vi "Set Calibration (SubVI).vi"(11 "Calibration in":T1 {"Max Current A" format="%#_g mA"; "Max Current B" format="%#_g mA"; "UCL A" format="%#_g mA"; "LCL A" format="%#_g mA"; "UCL B" format="%#_g mA"; "LCL B" format="%#_g mA"}) -> (1 "Array":string[](array[string]))   [LabVIEW 2015]
uses:
  03 Type Def & Global/Calibration.ctl
  <vilib>/Utility/miscctls.llb/LVPointTypeDef.ctl
panel:
  in  "Cancel Button":bool
  in  "OK Button":bool
  in  "Calibration":T1={"Max Current A"=290.0, "Max Current B"=290.0, "UCL A"=290.0, "UCL B"=290.0, "LCL A"=0.0, "LCL B"=0.0} {"Max Current A" format="%#_g mA"; "Max Current B" format="%#_g mA"; "UCL A" format="%#_g mA"; "LCL A" format="%#_g mA"; "UCL B" format="%#_g mA"; "LCL B" format="%#_g mA"}
  # "Please change the calbration values as needed"
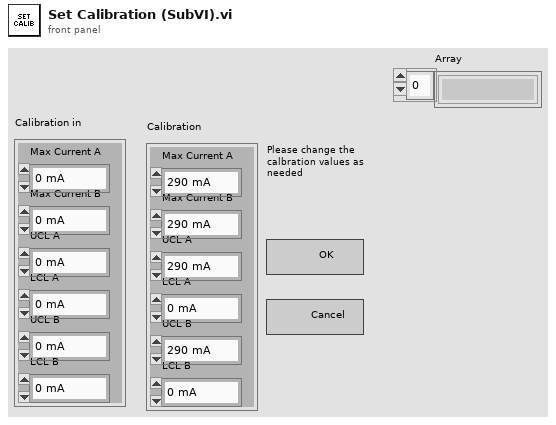
[diagram p1: front panel]
types:
  T1 = typedef "Calibration.ctl" = cluster{"Max Current A":dbl, "Max Current B":dbl, "UCL A":dbl, "UCL B":dbl, "LCL A":dbl, "LCL B":dbl}
  T2 = typedef "LVPointTypeDef.ctl" = cluster{"Horizontal":i16, "Vertical":i16}
  T3 = cluster{"Max Current A":bool, "Max Current B":bool, "UCL A":bool, "UCL B":bool, "LCL A":bool, "LCL B":bool}
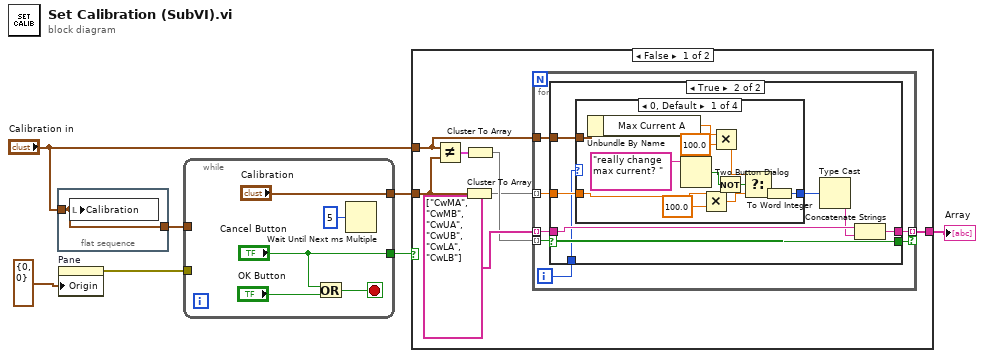
[diagram p0: block diagram]
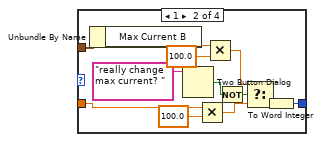
[diagram p3: hidden frame]
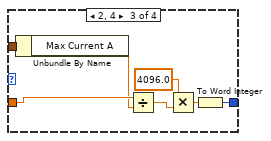
[diagram p4: hidden frame]
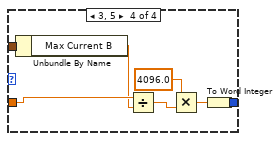
[diagram p5: hidden frame]
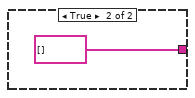
[diagram p6: hidden frame]
diagram:
  n1 = flat-sequence {
    tunnel: "Calibration in" -> [w8]
    tunnel: [w8] -> w1
    frame #0 {
      n2 = local write "Calibration"(w8) -> ()
    }
  }
  n3 = property on="Pane" class="Pane"("Origin"=T2 {"Horizontal"=0, "Vertical"=0}) -> (error out=w2:errorcluster)  [unwired: 2 in, 1 out]
  n4 = while {
    tunnel: ["Calibration"] -> w6
    tunnel: ["Cancel Button"] -> w5
    tunnel: w2 -> [_]
    tunnel: w1 -> [_]
    stop <- w13 stop-if-true
    n5 = Or(x="Cancel Button", y="OK Button") -> (x .or. y?=w13:bool)
    n6 = Wait Until Next ms Multiple(millisecond multiple=u32 5) -> ()  [unwired: 1 out]
  }
  n7 = case shown="False" w5 {
    tunnel: "Calibration in" -> [w14 _]
    tunnel: w6 -> [w16 _]
    tunnel: [w18 string[] []] -> w4
    frame False {
      n8 = Not Equal?(x=w14, y=w16) -> (x != y?=w17:T3)
      n9 = Cluster To Array(cluster=w16) -> (array=w15:dbl[])
      n10 = Cluster To Array(cluster=w17) -> (array=w19:bool[])
      n11 = for {
        tunnel: string[] ["CwMA", "CwMB", "CwUA", "CwUB", "CwLA", "CwLB"] -> [w25] mode=indexing
        tunnel: w19 -> [w27] mode=indexing
        tunnel: [w24] -> w18 mode=indexing if=w26
        tunnel: w15 -> [w23] mode=indexing
        tunnel: w14 -> [w21]
        i -> [w22]
        n12 = case shown="True" w27 {
          selector: w27 -> [w29 w37]
          tunnel: [w29 w37] -> w26
          tunnel: w25 -> [w28 w34]
          tunnel: [w28 w36] -> w24
          tunnel: w23 -> [_ w35]
          tunnel: w22 -> [_ w31]
          tunnel: w21 -> [_ w32]
          frame False {
          }
          frame True {
            n13 = case shown="0, Default" w31 {
              tunnel: w35 -> [w40 w52 w66 w73]
              tunnel: [w44 w56 w68 w75] -> w30
              tunnel: w32 -> [w48 w60 w67 w74]
              frame 0, Default {
                n14 = Unbundle By Name(w48) -> ("Max Current A"=w42:dbl)
                n15 = Two Button Dialog(message="really change max current? ") -> (T button?=w46:bool)  [unwired: 2 in]
                n16 = Multiply(x=w40, y=100.0) -> (x*y=w38:dbl)
                n17 = Multiply(x=w42, y=100.0) -> (x*y=w41:dbl)
                n18 = Not(x=w46) -> (.not. x?=w45:bool)
                n19 = Select(t=w41, s=w45, f=w38) -> (s? t:f=w47:dbl)
                n20 = To Word Integer(number=w47) -> (16bit integer=w44:i16)
              }
              frame 1 {
                n21 = Unbundle By Name(w60) -> ("Max Current B"=w54:dbl)
                n22 = Two Button Dialog(message="really change max current? ") -> (T button?=w58:bool)  [unwired: 2 in]
                n23 = Multiply(x=w52, y=100.0) -> (x*y=w50:dbl)
                n24 = Multiply(x=w54, y=100.0) -> (x*y=w53:dbl)
                n25 = Not(x=w58) -> (.not. x?=w57:bool)
                n26 = Select(t=w53, s=w57, f=w50) -> (s? t:f=w59:dbl)
                n27 = To Word Integer(number=w59) -> (16bit integer=w56:i16)
              }
              frame 2, 4 {
                n28 = Unbundle By Name(w67) -> ("Max Current A"=w65:dbl)
                n29 = Divide(x=w66, y=w65) -> (x/y=w63:dbl)
                n30 = Multiply(x=4096.0, y=w63) -> (x*y=w64:dbl)
                n31 = To Word Integer(number=w64) -> (16bit integer=w68:i16)
              }
              frame 3, 5 {
                n32 = Unbundle By Name(w74) -> ("Max Current B"=w72:dbl)
                n33 = Divide(x=w73, y=w72) -> (x/y=w70:dbl)
                n34 = Multiply(x=4096.0, y=w70) -> (x*y=w71:dbl)
                n35 = To Word Integer(number=w71) -> (16bit integer=w75:i16)
              }
            }
            n36 = Type Cast(x=w30) -> (*(type *) &x=w33:string)  [unwired: 1 in]
            n37 = Concatenate Strings(w34, w33) -> (w36:string)
          }
        }
      }
    }
    frame True {
    }
  }
  "Array" <- w4
